vi "merge_Accumulate.vi"   [LabVIEW 2017, in "NI_FunctionBlockMergeVIs.lvlib"]
doc: "Accumulates a point-by-point sum. When <B>enable</B> is TRUE, this function block adds the value of <B>input</B> to the value of <B>accumulation</B>."
uses:
  <vilib>/functionblocks/NI_FunctionBlockMergeVIs.lvlib
  <vilib>/functionblocks/FB Core/FB Core.xnode
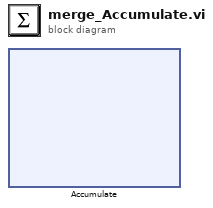
[diagram p0: block diagram]
diagram:
  n1 = xnode "Accumulate"() -> ()  [unwired: 4 in, 2 out]
